vi "Build Behavior.vi"(8 "error in (no error)":errorcluster, 11 "Control Builder in":refnum<class "GUI Control Builder.lvclass">) -> (0 "error out":errorcluster, 2 "Panel Request Behavior":refnum<class "Panel Behavior.lvclass">, 3 "Control Builder out":refnum<class "GUI Control Builder.lvclass">)   [LabVIEW 2015, in "GUI Control Builder.lvclass"]
uses:
  GUI Control Builder.lvclass
  _Depences/Panel API/Panel Request/Panle Requeset Behavior/Panel Behavior.lvclass
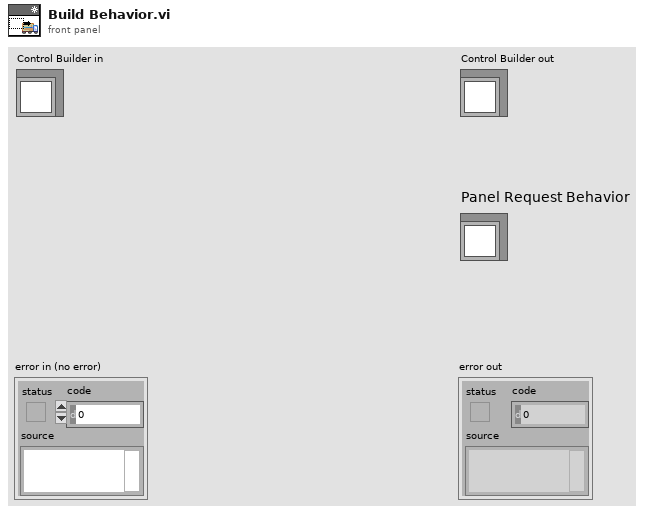
[diagram p1: front panel]
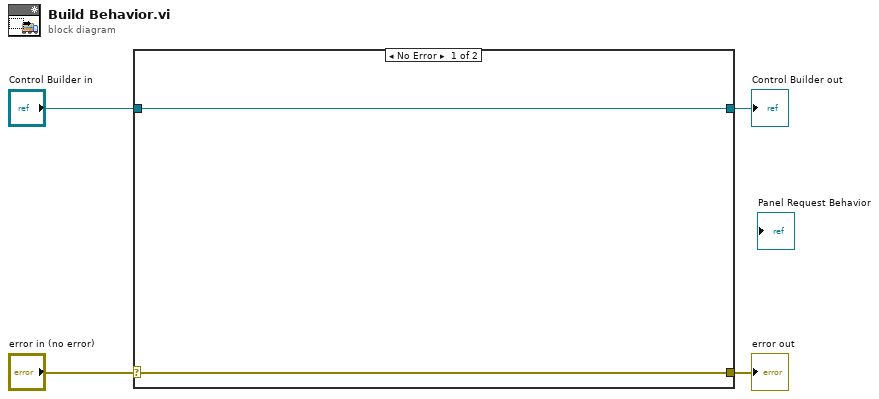
[diagram p0: block diagram]
diagram:
  n1 = case shown="No Error" "error in (no error)" {
    selector: "error in (no error)" -> [w5 w8]
    tunnel: [w5 w8] -> w3
    tunnel: [w6 w7] -> w1
    tunnel: "Control Builder in" -> [w6 w7]
    frame No Error {
    }
    frame Error {
    }
  }
  "error out" <- w3
  "Control Builder out" <- w1
